vi "Swerve Sensors Open.vi"(8 "Rear Left Wheel":T4, 9 "Rear Right Wheel":T4, 10 "Front Left Wheel":T4, 11 "Front Right Wheel":T4) -> (2 "Swerve Sensors DevRef":T1)   [LabVIEW 2014]
uses:
  <vilib>/Rock Robotics/SystemInterfaces/AI/FPGA_AIChannel.ctl
  Swerve Sensors DevRef.ctl
  <vilib>/Rock Robotics/WPI/AnalogChannel/WPI_AnalogChannelDevRef.ctl
  <vilib>/Rock Robotics/SystemInterfaces/Typedef/FPGA_TypedefAnalogModule.ctl
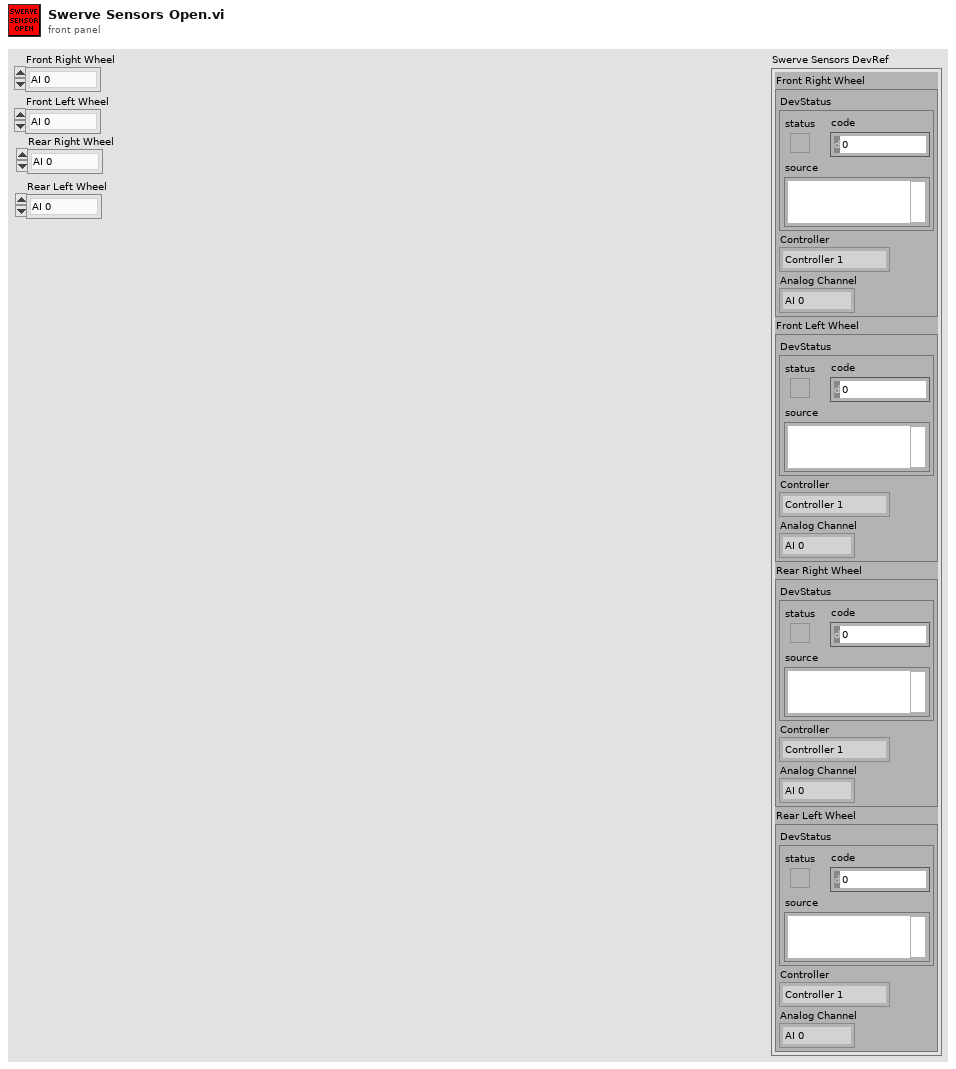
[diagram p1: front panel]
types:
  T1 = typedef "Swerve Sensors DevRef.ctl" = cluster{"Front Right Wheel":T2, "Front Left Wheel":T2, "Rear Right Wheel":T2, "Rear Left Wheel":T2}
  T2 = typedef "WPI_AnalogChannelDevRef.ctl" = cluster{"DevStatus":errorcluster, "Controller":T3, "Analog Channel":T4}
  T3 = typedef "FPGA_TypedefAnalogModule.ctl" = enum16{"Controller 1"}
  T4 = typedef "FPGA_AIChannel.ctl" = enum8{"AI 0", "AI 1", "AI 2", "AI 3", "AI MXP 0", "AI MXP 1", "AI MXP 2", "AI MXP 3", "Invalid"}
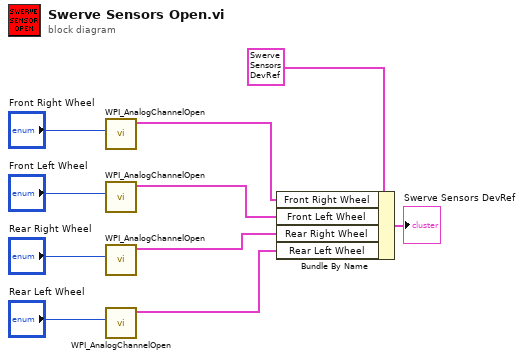
[diagram p0: block diagram]
diagram:
  n1 = call <vilib>:"WPI_AnalogChannelOpen.vi"("Analog Channel"="Front Right Wheel") -> ("AIDeviceRef"=w5:T2)  [unwired: 9 in, 1 out]
  n2 = call <vilib>:"WPI_AnalogChannelOpen.vi"("Analog Channel"="Front Left Wheel") -> ("AIDeviceRef"=w4:T2)  [unwired: 9 in, 1 out]
  n3 = call <vilib>:"WPI_AnalogChannelOpen.vi"("Analog Channel"="Rear Right Wheel") -> ("AIDeviceRef"=w3:T2)  [unwired: 9 in, 1 out]
  n4 = call <vilib>:"WPI_AnalogChannelOpen.vi"("Analog Channel"="Rear Left Wheel") -> ("AIDeviceRef"=w2:T2)  [unwired: 9 in, 1 out]
  n5 = Bundle By Name(cluster=T1 {"Front Right Wheel"={"DevStatus"={"status"=FALSE, "code"=0, "source"=""}, "Controller"=enum."Controller 1", "Analog Channel"=enum."AI 0"}, "Front Left Wheel"={"DevStatus"={"status"=FALSE, "code"=0, "source"=""}, "Controller"=enum."Controller 1", "Analog Channel"=enum."AI 0"}, "Rear Right Wheel"={"DevStatus"={"status"=FALSE, "code"=0, "source"=""}, "Controller"=enum."Controller 1", "Analog Channel"=enum."AI 0"}, "Rear Left Wheel"={"DevStatus"={"status"=FALSE, "code"=0, "source"=""}, "Controller"=enum."Controller 1", "Analog Channel"=enum."AI 0"}}, "Front Right Wheel"=w5, "Front Left Wheel"=w4, "Rear Right Wheel"=w3, "Rear Left Wheel"=w2) -> (→"Swerve Sensors DevRef":T1)
